vi "GlbCamHndls.vi"() -> ()   [LabVIEW 2010]
panel:
  in  "Y dimension":u32
  in  "X dimension":u32
  out "spectrometers  opened":bool[](array[boolean])
  in  "Number of spectrometers opened":u32
  in  "Spectrometer Handles":u32[](array[numeric])
  out "camera opened":bool[](array[boolean])
  in  "Number of cameras opened":u32
  in  "Camera Handles":u32[](array[numeric])
  # "Gloabal vairables for camara and spectrometer"
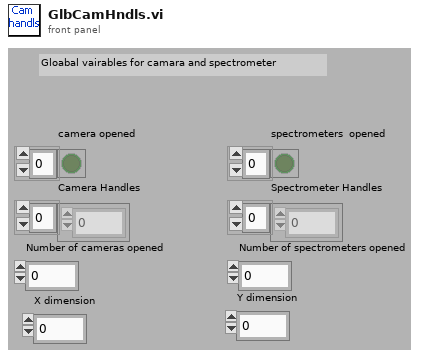
[diagram p1: front panel]
diagram:
